vi "Unflatten Value.vi"(8 "error in (no error)":errorcluster, 10 "Value":string, 11 "Boolean in":refnum<class "Double.lvclass">) -> (0 "error out":errorcluster, 3 "Boolean out":refnum<class "Double.lvclass">)   [LabVIEW 2019, in "Double.lvclass"]
uses:
  <vilib>/gpm_packages/@cs/data-type-serializer/source/Double/Double.lvclass
  <vilib>/gpm_packages/@cs/data-type-serializer/source/Double/Double.lvclass/Double.ctl
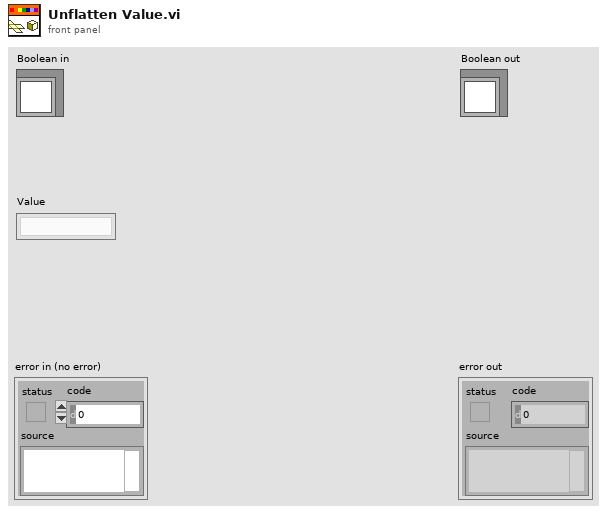
[diagram p1: front panel]
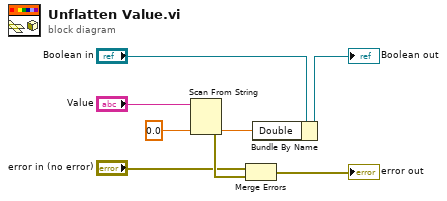
[diagram p0: block diagram]
diagram:
  n1 = Scan From String(input string="Value", default 1=0.0) -> (error out=w6:errorcluster, output 1=w5:dbl)  [unwired: 3 in, 2 out]
  n2 = Merge Errors("error in (no error)", w6) -> (→"error out":errorcluster)
  n3 = Bundle By Name(cluster="Boolean in", "Double"=w5) -> (→"Boolean out":refnum<class "Double.lvclass">)
